vi "TrapPower.vi"() -> ()   [LabVIEW 2016]
uses:
  <vilib>/Analysis/baseanly.llb/Mean (DBL).vi
  <vilib>/express/express analysis/Spectral/Block/exnSpectralBlock spectral measurements PSD poly.vi
  <vilib>/express/express analysis/Spectral/Block/exnSpectralBlock spectral measurements PSD DDT.vi
  <vilib>/express/express analysis/Spectral/XNode/ExpressSpectralMeasurementsBlockNode.xnode
  <vilib>/Analysis/NI_AALBase.lvlib
panel:
  out "# in queue":i32
  in  "stop":bool
  out "B1X PSD":dynamicdata(graph)
  out "B1X":dbl(graph)
  in  "Vin 2":dbl=1.0 min=1.0 max=10.0
  in  "stop 2":bool
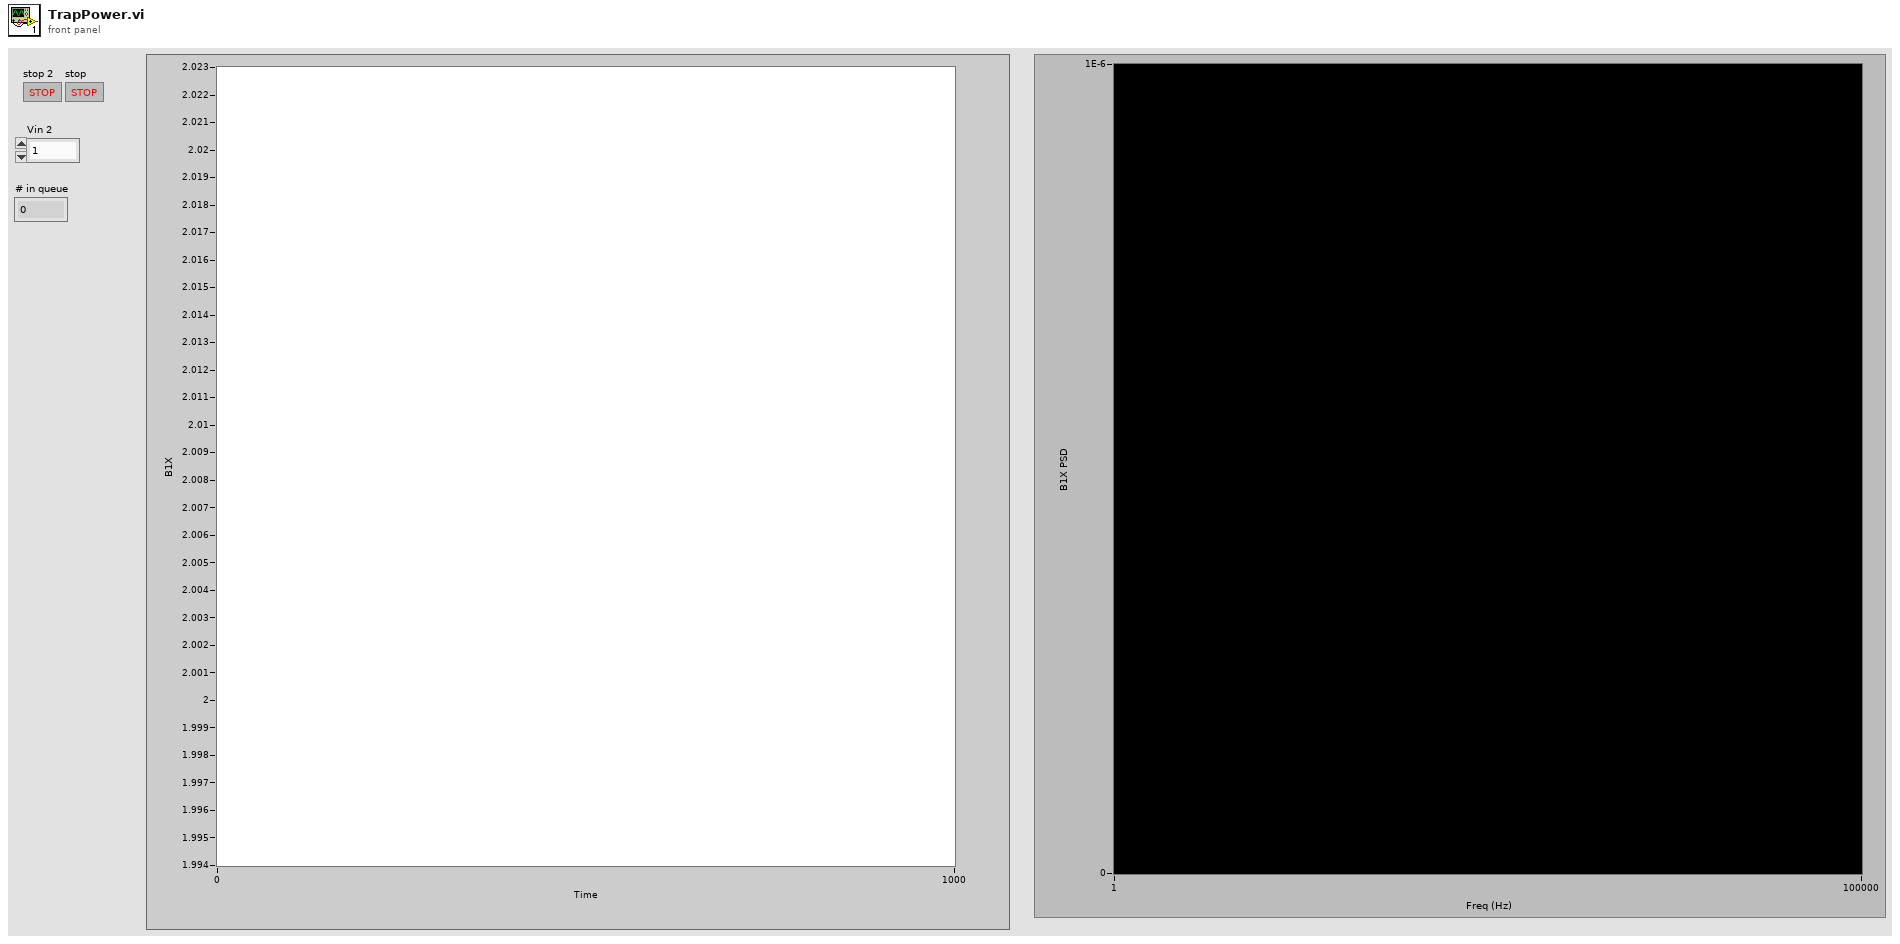
[diagram p1: front panel]
types:
  T1 = cluster{"averaging mode":u16, "weighting mode":u16, "number of averages":u32}
  T2 = cluster{"dB On (F)":bool, "unwrap phase (F)":bool, "convert to degree (F)":bool}
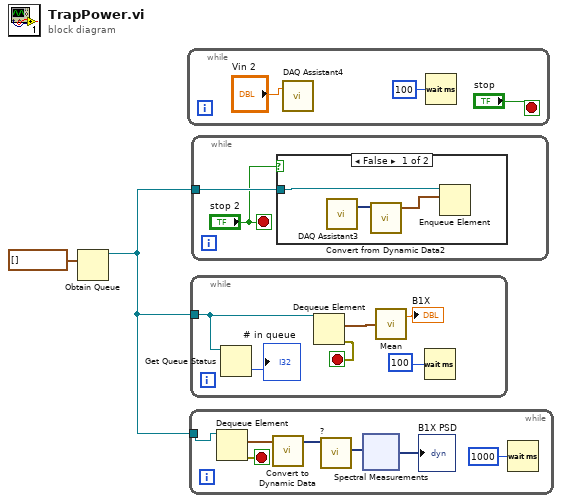
[diagram p0: block diagram]
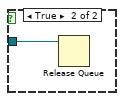
[diagram p2: hidden frame]
diagram:
  n1 = Obtain Queue(element data type=waveform(sgl)[] []) -> (queue out=w1:refnum<queue>)  [unwired: 4 in, 2 out]
  n2 = while {
    stop <- "stop" stop-if-true
    n3 = call "DAQ Assistant4"("data"="Vin 2") -> ()  [unwired: 17 in, 2 out]
    n4 = Wait (ms)(milliseconds to wait=u32 100) -> ()  [unwired: 1 out]
  }
  n5 = while {
    tunnel: w1 -> [w8]
    stop <- w6 stop-if-true
    n6 = Dequeue Element(queue=w8) -> (element=w7:waveform(sgl)[], error out=w6:errorcluster)  [unwired: 2 in, 2 out]
    n7 = call "Convert to Dynamic Data"("Array of Waveforms"=w7) -> ("Dynamic Data Type"=w11:dynamicdata)  [unwired: 3 in]
    n8 = call "?"("Signals"=w11) -> ("Collected Signals"=w12:dynamicdata)  [unwired: 9 in, 1 out]
    n9 = xnode ("Spectral Measurements")("Signals"=w12) -> ("PSD"=→"B1X PSD":dynamicdata)  [unwired: 2 in, 2 out]
    n10 = Wait (ms)(milliseconds to wait=u32 1000) -> ()  [unwired: 1 out]
  }
  n11 = while {
    tunnel: w1 -> [w23]
    stop <- w28 stop-if-true
    n12 = Get Queue Status(queue=w23) -> (# elements in queue=→"# in queue":i32)  [unwired: 2 in, 7 out]
    n13 = Dequeue Element(queue=w23) -> (element=w27:waveform(sgl)[], error out=w28:errorcluster)  [unwired: 2 in, 2 out]
    n14 = call-poly <vilib>:"Mean.vi"("X"=w27) -> ("mean"=→"B1X":dbl)  [unwired: 1 out]
    n15 = Wait (ms)(milliseconds to wait=u32 100) -> ()  [unwired: 1 out]
  }
  n16 = while {
    tunnel: w1 -> [w30]
    stop <- "stop 2" stop-if-true
    n17 = case shown="False" "stop 2" {
      tunnel: w30 -> [w31 w34]
      frame False {
        n18 = call "DAQ Assistant3"() -> ("data"=w33:dynamicdata)  [unwired: 16 in, 3 out]
        n19 = call "Convert from Dynamic Data2"("Dynamic Data Type"=w33) -> ("Array of Waveform"=w32:waveform(dbl)[])  [unwired: 3 in]
        n20 = Enqueue Element(queue=w31, element=w32) -> ()  [unwired: 2 in, 3 out]
      }
      frame True {
        n21 = Release Queue(queue=w34) -> ()  [unwired: 2 in, 3 out]
      }
    }
  }
